vi "Read getAll.vi"(8 "error in (no error)":errorcluster, 11 "instrument.PPMS in":refnum<class "instrument.PPMS.lvclass">) -> (0 "error out":errorcluster, 2 "getAll":T1, 3 "instrument.PPMS out":refnum<class "instrument.PPMS.lvclass">)   [LabVIEW 2019, in "instrument.PPMS.lvclass"]
uses:
  instrument.PPMS.lvclass
  Typedefs/PPMS.getAll--cluster.ctl
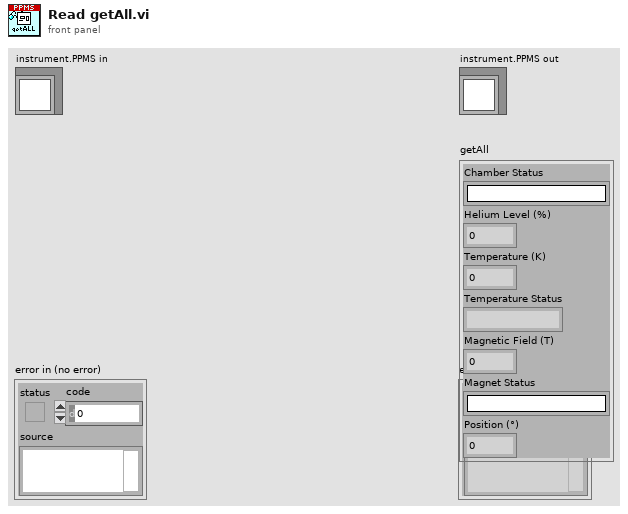
[diagram p1: front panel]
types:
  T1 = typedef "instrument.PPMS.lvclass/PPMS.getAll--cluster.ctl" = cluster{"Chamber Status":string, "Helium Level (%)":dbl, "Temperature (K)":dbl, "Temperature Status":string, "Magnetic Field (T)":dbl, "Magnet Status":string, "Position (°)":dbl}
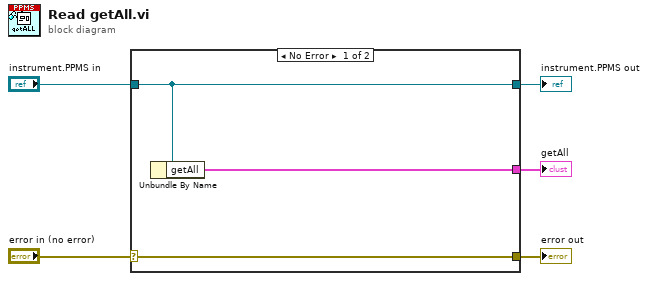
[diagram p0: block diagram]
diagram:
  n1 = case shown="No Error" "error in (no error)" {
    selector: "error in (no error)" -> [w8 w9]
    tunnel: [w8 w9] -> w4
    tunnel: [w7 w10] -> w2
    tunnel: "instrument.PPMS in" -> [w7 w10]
    tunnel: [w6 _] -> w1
    frame No Error {
      n2 = Unbundle By Name(w7) -> ("getAll"=w6:T1)
    }
    frame Error {
    }
  }
  "error out" <- w4
  "instrument.PPMS out" <- w2
  "getAll" <- w1
